vi "Array TDX to Script TDX(SubVI).vi"(11 "TDX IN":bool[](array[boolean])) -> (3 "TDX CONFIG":string[](array[string]))   [LabVIEW 2014, in "CAP-USB.lvlib"]
doc: "TOMA EL ARRAY DE TRANSDUCTORES QUE ELIGE ELIGE EL OPERARIO Y LO TRANSFORMA EN LAS LINEAS DE COMANDO NECESARIAS PARA ARMAR EL SCRIPT EN LA PLACA"
uses:
  CAP-USB.lvlib
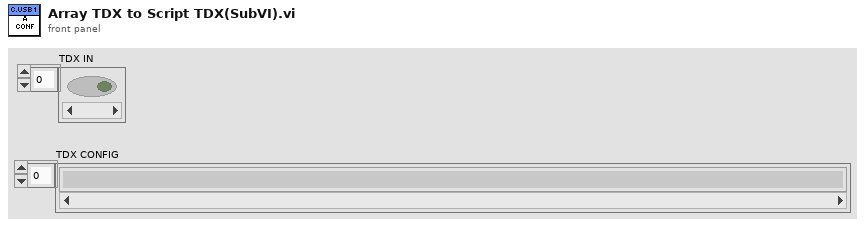
[diagram p1: front panel]
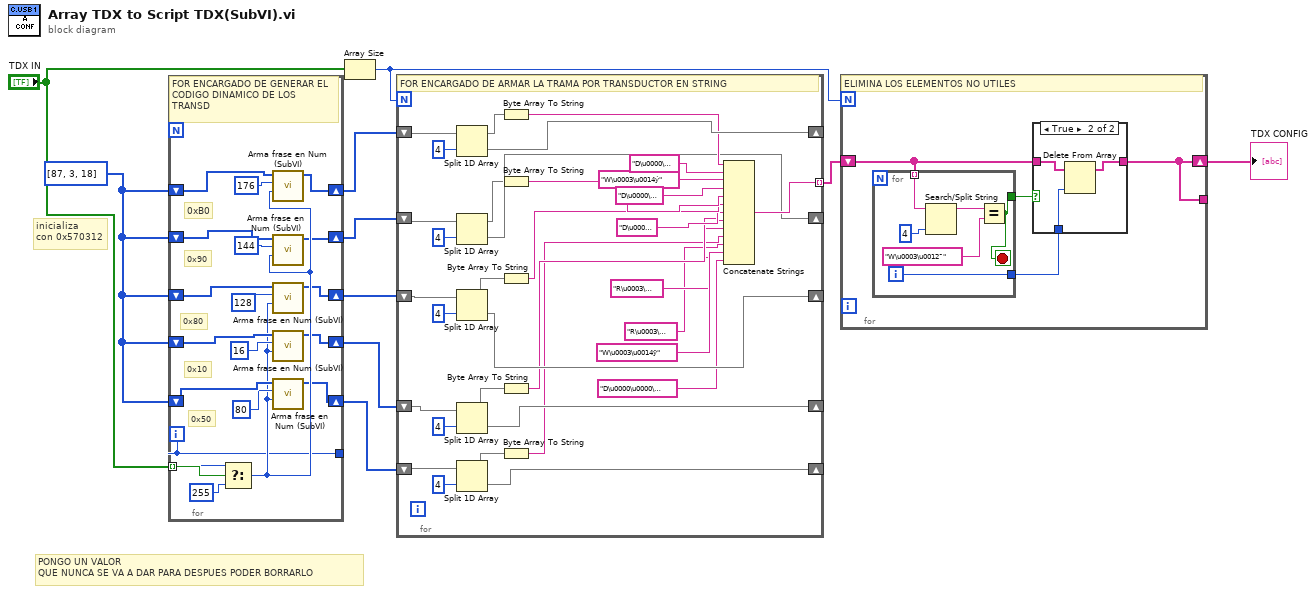
[diagram p0: block diagram]
diagram:
  w9 = u8[] [87, 3, 18]
  # "PONGO UN VALOR \nQUE NUNCA SE VA A DAR PARA DESPUES PODER BORRARLO"
  # "inicializa\ncon 0x570312"
  n1 = for {
    tunnel: "TDX IN" -> [w29] mode=indexing
    shift-right: [w16] -> w10
    shift-left: w9 -> [w27]
    shift-right: [w15] -> w8
    shift-left: w9 -> [w24]
    shift-right: [w14] -> w7
    shift-left: w9 -> [w23]
    shift-right: [w13] -> w6
    shift-left: w9 -> [w22]
    shift-right: [w12] -> w5
    shift-left: w9 -> [w21]
    tunnel: [w11] -> _
    i -> [w11]
    # "0x50"
    # "0x10"
    # "0x80"
    # "0x90"
    # "0xB0"
    # "FOR ENCARGADO DE GENERAR EL CODIGO DINAMICO DE LOS TRANSD"
    n2 = Select(t=w11, s=w29, f=255) -> (s? t:f=w17:i32)
    n3 = call "Arma frase en Num (SubVI).vi"("Posicion"=w17, "Direccion"=176, "Codigo"=w27) -> ("Codigo Completa"=w16:u8[])  [unwired: 8 in]
    n4 = call "Arma frase en Num (SubVI).vi"("Posicion"=w17, "Direccion"=144, "Codigo"=w24) -> ("Codigo Completa"=w15:u8[])  [unwired: 8 in]
    n5 = call "Arma frase en Num (SubVI).vi"("Posicion"=w17, "Direccion"=128, "Codigo"=w23) -> ("Codigo Completa"=w14:u8[])  [unwired: 8 in]
    n6 = call "Arma frase en Num (SubVI).vi"("Posicion"=w17, "Direccion"=16, "Codigo"=w22) -> ("Codigo Completa"=w13:u8[])  [unwired: 8 in]
    n7 = call "Arma frase en Num (SubVI).vi"("Posicion"=w17, "Direccion"=80, "Codigo"=w21) -> ("Codigo Completa"=w12:u8[])  [unwired: 8 in]
  }
  n8 = Array Size(array="TDX IN") -> (size(s)=w1:i32)
  n9 = for {
    N: w1 -> [_]
    shift-right: [w60] -> _
    shift-left: w10 -> [w63]
    tunnel: [w58] -> w4 mode=indexing
    shift-right: [w57] -> _
    shift-left: w8 -> [w55]
    shift-right: [w52] -> _
    shift-left: w7 -> [w54]
    shift-right: [w51] -> _
    shift-left: w6 -> [w49]
    shift-right: [w46] -> _
    shift-left: w5 -> [w48]
    # "FOR ENCARGADO DE ARMAR LA TRAMA POR TRANSDUCTOR EN STRING"
    n10 = Split 1D Array(array=w63, index=4) -> (first subarray=w61:u8[], second subarray=w60:u8[])
    n11 = Split 1D Array(array=w55, index=4) -> (first subarray=w45:u8[], second subarray=w57:u8[])
    n12 = Split 1D Array(array=w54, index=4) -> (first subarray=w44:u8[], second subarray=w52:u8[])
    n13 = Split 1D Array(array=w49, index=4) -> (first subarray=w43:u8[], second subarray=w51:u8[])
    n14 = Split 1D Array(array=w48, index=4) -> (first subarray=w42:u8[], second subarray=w46:u8[])
    n15 = Byte Array To String(unsigned byte array=w61) -> (string=w59:string)
    n16 = Byte Array To String(unsigned byte array=w45) -> (string=w36:string)
    n17 = Byte Array To String(unsigned byte array=w44) -> (string=w35:string)
    n18 = Byte Array To String(unsigned byte array=w43) -> (string=w33:string)
    n19 = Byte Array To String(unsigned byte array=w42) -> (string=w31:string)
    n20 = Concatenate Strings(w59, "D\u0000\u0000\u0000\u0014", "W\u0003\u0014ý", "D\u0000\u0000\u0000\u0002", w36, w35, "D\u0000\u0000\u0000\u0014", w33, "R\u0003\u0010", w31, "R\u0003\u0010", "W\u0003\u0014ÿ", "D\u0000\u0000\u0000\u0014") -> (w58:string)
  }
  n21 = for {
    N: w1 -> [_]
    shift-right: [w66] -> w3
    shift-left: w4 -> [w65]
    tunnel: [w66] -> _
    # "ELIMINA LOS ELEMENTOS NO UTILES"
    n22 = for {
      tunnel: [w68] -> w67
      tunnel: w65 -> [w70] mode=indexing
      tunnel: [w69] -> w64
      i -> [w69]
      stop <- w68 stop-if-true
      n23 = Search/Split String(string=w70, offset (0)=4) -> (substring before match=w72:string)  [unwired: 1 in, 2 out]
      n24 = Equal?(x=w72, y="W\u0003\u0012¯") -> (x = y?=w68:bool)
    }
    n25 = case shown="True" w67 {
      tunnel: w65 -> [w74 w77]
      tunnel: [w74 w76] -> w66
      tunnel: w64 -> [_ w75]
      frame False {
      }
      frame True {
        n26 = Delete From Array(array=w77, index=w75) -> (array with subset deleted=w76:string[])  [unwired: 1 in, 1 out]
      }
    }
  }
  "TDX CONFIG" <- w3
